vi "Get Lock.vi"(8 "error in (no error)":errorcluster, 11 "SQLite3LV Cursor in":refnum<class "cursor.lvclass">) -> (0 "error out":errorcluster, 2 "sqlite lock":refnum<data-value>, 3 "SQLite3LV Cursor out":refnum<class "cursor.lvclass">)   [LabVIEW 2014, in "SQLite3LV.lvlib" / "cursor.lvclass"]
doc: "Returns the lock object associated with the database connection.\n\nClient code is required to implement all synchronization to ensure that the database connection is used by only one thread at a time. \n\nThe helper methods \"Get Lock\" will return a memory reference lock for the database connection. This lock may be use to synchronize access to the database connection from multiple threads or subVIs."
uses:
  cursor.lvclass
  cursor.lvclass/cursor.ctl
  SQLite3 Class/sqlite3.lvclass
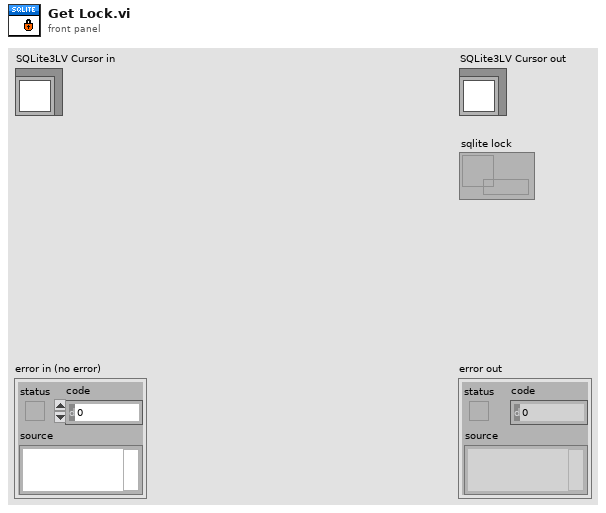
[diagram p1: front panel]
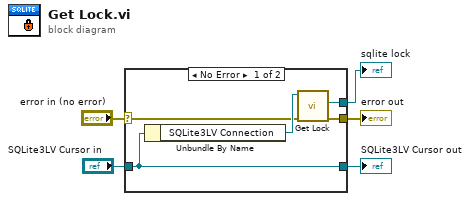
[diagram p0: block diagram]
diagram:
  n1 = case shown="No Error" "error in (no error)" {
    selector: "error in (no error)" -> [w8 w12]
    tunnel: [w7 w12] -> w4
    tunnel: [w10 w11] -> w2
    tunnel: "SQLite3LV Cursor in" -> [w10 w11]
    tunnel: [w6 _] -> w1
    frame No Error {
      n2 = Unbundle By Name(w10) -> ("SQLite3LV Connection"=w9:refnum<class "sqlite3.lvclass">)
      n3 = call "Get Lock.vi"("error in (no error)"=w8, "SQLite3LV Connection in"=w9) -> ("error out"=w7:errorcluster, "sqlite lock"=w6:refnum<data-value>)  [unwired: 7 in, 1 out]
    }
    frame Error {
    }
  }
  "error out" <- w4
  "SQLite3LV Cursor out" <- w2
  "sqlite lock" <- w1
